vi "Compute.vi"(8 "error in (no error)":errorcluster, 9 "Operation":T1, 10 "Operand2":string, 11 "Operand1":string) -> (0 "error out":errorcluster, 3 "Result":string)   [LabVIEW 2021]
uses:
  Operation.ctl
  <vilib>/Utility/error.llb/Error Cluster From Error Code.vi
  <vilib>/ErrorRing/Error Ring.xnode
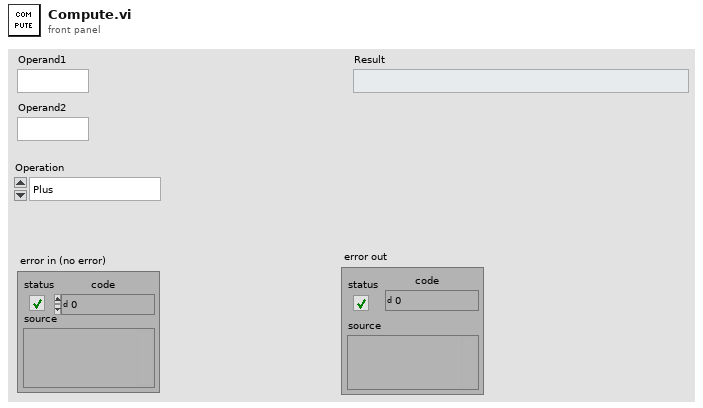
[diagram p1: front panel]
types:
  T1 = typedef "Operation.ctl" = enum16{"Plus", "Minus", "Multiply", "Divide"}
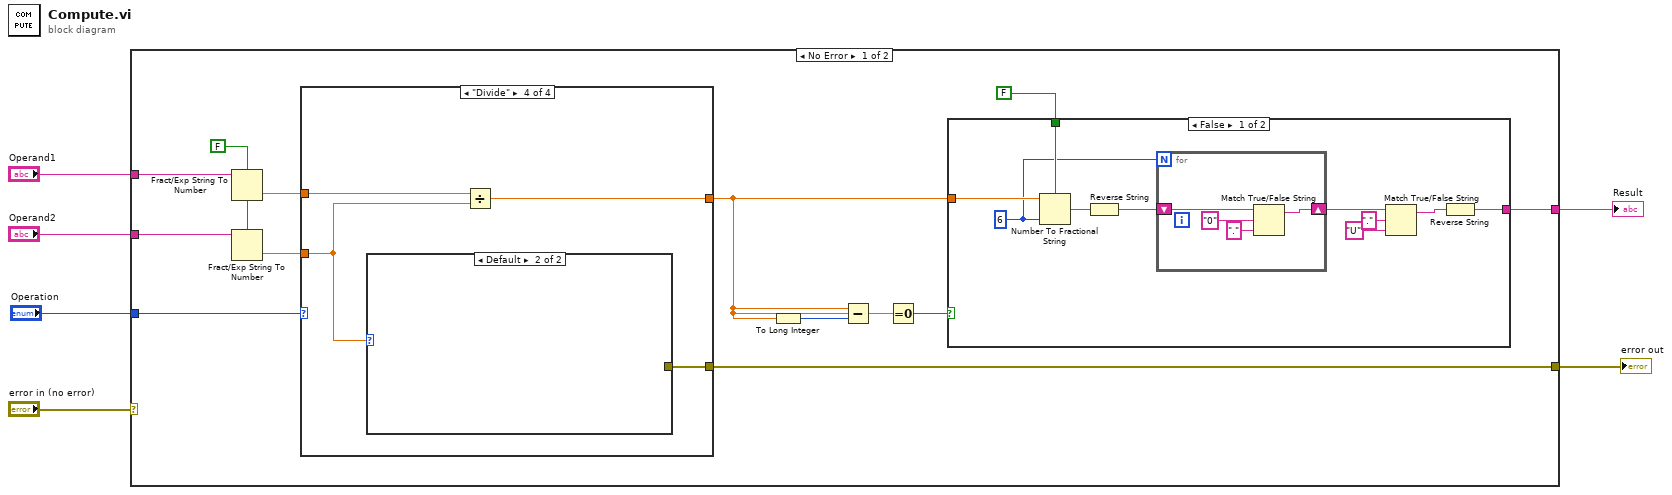
[diagram p0: block diagram]
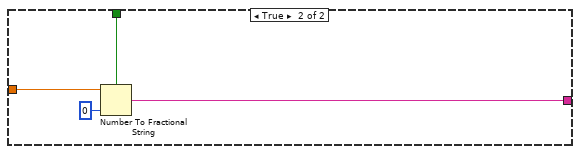
[diagram p2: hidden frame]
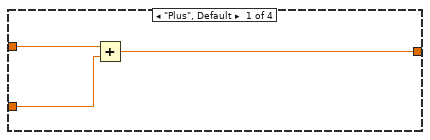
[diagram p3: hidden frame]
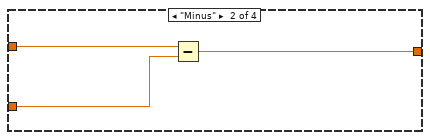
[diagram p4: hidden frame]
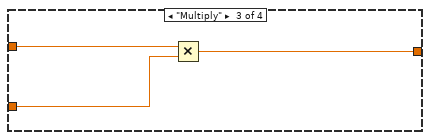
[diagram p5: hidden frame]
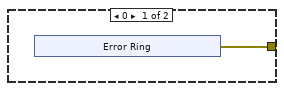
[diagram p6: hidden frame]
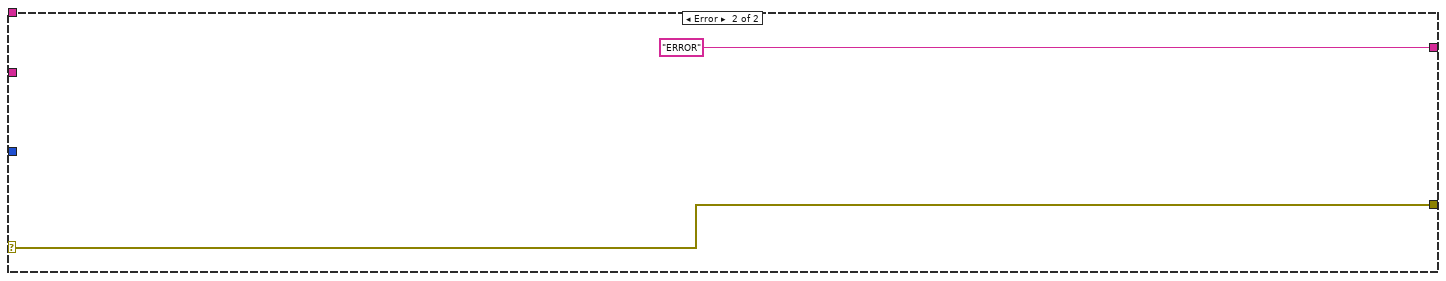
[diagram p7: hidden frame]
diagram:
  n1 = case shown="No Error" "error in (no error)" {
    selector: "error in (no error)" -> [_ w57]
    tunnel: [w7 w57] -> w5
    tunnel: "Operand1" -> [w18 _]
    tunnel: "Operand2" -> [w17 _]
    tunnel: "Operation" -> [w16 _]
    tunnel: [w9 "ERROR"] -> w1
    frame No Error {
      w12 = FALSE ("use system decimal point (T)")
      n2 = Fract/Exp String To Number(use system decimal point (T)=w12, string=w18) -> (number=w15:dbl)  [unwired: 2 in, 1 out]
      n3 = Fract/Exp String To Number(use system decimal point (T)=w12, string=w17) -> (number=w14:dbl)  [unwired: 2 in, 1 out]
      n4 = case shown="\"Divide\"" w16 {
        tunnel: w15 -> [w39 w42 w45 w49]
        tunnel: w14 -> [w38 w41 w44 w47]
        tunnel: [w37 w40 w43 w48] -> w11
        tunnel: [_ _ _ w46] -> w7
        frame "Plus", Default {
          n5 = Add(x=w39, y=w38) -> (x+y=w37:dbl)
        }
        frame "Minus" {
          n6 = Subtract(x=w42, y=w41) -> (x-y=w40:dbl)
        }
        frame "Multiply" {
          n7 = Multiply(x=w45, y=w44) -> (x*y=w43:dbl)
        }
        frame "Divide" {
          n8 = case shown="Default" w47 {
            tunnel: [w50 _] -> w46
            frame 0 {
              n9 = xnode "Error Ring"() -> ("error out"=w50:errorcluster)
            }
            frame Default {
            }
          }
          n10 = Divide(x=w49, y=w47) -> (x/y=w48:dbl)
        }
      }
      n11 = To Long Integer(number=w11) -> (32bit integer=w13:i32)
      n12 = Subtract(x=w11, y=w13) -> ()  [unwired: 1 out]
      n13 = Equal To 0?(x=w11) -> (x = 0?=w8:bool)
      n14 = case shown="False" w8 {
        tunnel: w11 -> [w28 w36]
        tunnel: FALSE ("use system decimal point (T)") -> [w27 w34]
        tunnel: [w25 w33] -> w9
        frame False {
          w26 = i16 6 ("precision (6)")
          n15 = Number To Fractional String(use system decimal point (T)=w27, number=w28, precision (6)=w26) -> (F-format string=w24:string)  [unwired: 1 in]
          n16 = Reverse String(1:w24) -> (0:w23:string)
          n17 = for {
            N: w26 -> [_]
            shift-right: [w29] -> w22
            shift-left: w23 -> [w30]
            n18 = Match True/False String(2:"." ("false string"), 3:"0" ("true string"), 4:w30) -> (1:w29:string)  [unwired: 1 out]
          }
          n19 = Match True/False String(2:"U" ("false string"), 3:"." ("true string"), 4:w22) -> (1:w19:string)  [unwired: 1 out]
          n20 = Reverse String(1:w19) -> (0:w25:string)
        }
        frame True {
          n21 = Number To Fractional String(use system decimal point (T)=w34, number=w36, precision (6)=i16 0) -> (F-format string=w33:string)  [unwired: 1 in]
        }
      }
    }
    frame Error {
    }
  }
  "Result" <- w1
  "error out" <- w5
